vi "NameMapping_write.vi"(8 "error in (no error)":errorcluster, 11 "AE-NamesMapping":T1(array[cluster])=[{"AE-Name(Raw)"="Krčil, Pavel", "AE-Name (Proper)"="Pavel Krcil"}, {"AE-Name(Raw)"="Koretz, Martin", "AE-Name (Proper)"="Martin Koretz "}, {"AE-Name(Raw)"="Kuba, Ondrej", "AE-Name (Proper)"="Ondrej Kuba"}, {"AE-Name(Raw)"="Jadrný, Michal", "AE-Name (Proper)"="Michal Jadrny"}, {"AE-Name(Raw)"="Borzási, Dániel", "AE-Name (Proper)"="Daniel Borzasi"}, {"AE-Name(Raw)"="Przystawski, Sebastian", "AE-Name (Proper)"="Sebastian Przystawski"}, {"AE-Name(Raw)"="Stępień, Adriana Eleonora", "AE-Name (Proper)"="Adriana Stepien"}, {"AE-Name(Raw)"="Loska, Mateusz Piotr", "AE-Name (Proper)"="Mateusz Loska"}, {"AE-Name(Raw)"="Stavila, Denis", "AE-Name (Proper)"="Denis Stavila"}, {"AE-Name(Raw)"="Lipták, Jozef", "AE-Name (Proper)"="Jozef Liptak"}, {"AE-Name(Raw)"="Fülöp, Dániel", "AE-Name (Proper)"="Daniel Fulop"}, {"AE-Name(Raw)"="Balauta, Bogdan-Alexandru", "AE-Name (Proper)"="Bogdan Balauta"}, {"AE-Name(Raw)"="Curatu, Rares", "AE-Name (Proper)"="Rares Curatu"}, {"AE-Name(Raw)"="Kamińska, Katarzyna Małgorzata", "AE-Name (Proper)"="Katarzyna Kaminska"}]) -> (0 "error out":errorcluster)   [LabVIEW 2018, in "MainFrameLib.lvlib"]
uses:
  MainFrameLib.lvlib
  <vilib>/Utility/file.llb/Write Delimited Spreadsheet (string).vi
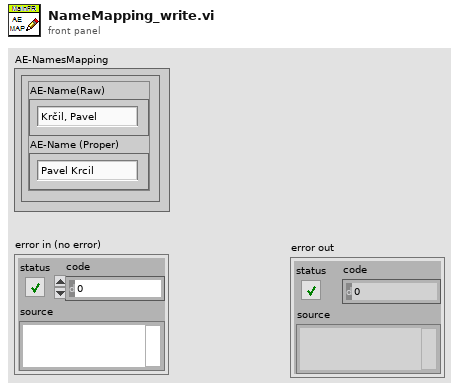
[diagram p1: front panel]
types:
  T1 = cluster{"AE-Name(Raw)":string, "AE-Name (Proper)":string}[]
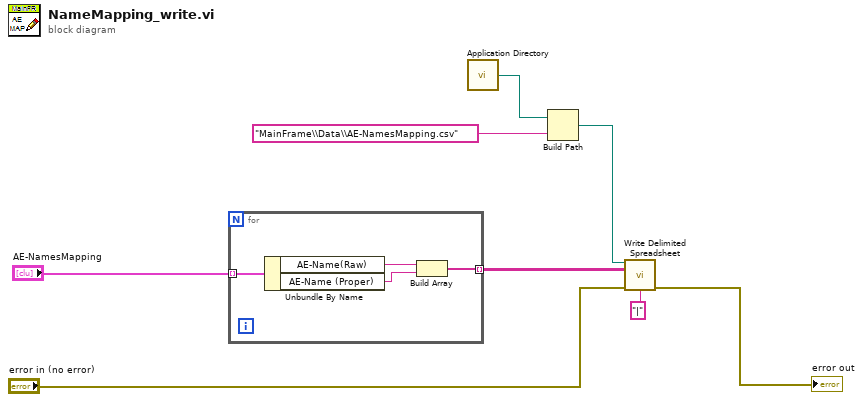
[diagram p0: block diagram]
diagram:
  n1 = for {
    tunnel: "AE-NamesMapping" -> [w12] mode=indexing
    tunnel: [w9] -> w4 mode=indexing
    n2 = Unbundle By Name(w12) -> ("AE-Name(Raw)"=w11:string, "AE-Name (Proper)"=w10:string)
    n3 = Build Array(w11, w10) -> (w9:string[])
  }
  n4 = call <vilib>:"Application Directory.vi"() -> ("Application Directory"=w8:path)
  n5 = Build Path(base path=w8, name or relative path="MainFrame\\Data\\AE-NamesMapping.csv") -> (appended path=w6:path)
  n6 = call-poly <vilib>:"Write Delimited Spreadsheet.vi"("file path (dialog if empty)"=w6, "2D data"=w4, "error in (no error)"="error in (no error)", "delimiter (\\t)"="|" ("delimiter (\\t)")) -> ("error out"=→"error out":errorcluster)  [unwired: 10 in, 1 out]
